vi "start.vi"() -> ()   [LabVIEW 2018]
uses:
  <vilib>/picture/picture.llb/imagedata.ctl
  SerialGlobal.vi
panel:
  out "Loop counts":i32
  out "ScanCode":i16
  out "NewVal":string
  out "Key":string
  in  "hum_pos":cluster{"pos.x":i32, "pos.y":i32}
  out "Main path":path
  out "image array":T1[](array[typedef])
  out "picture":picture
  out "status array":u8[][](array[numeric])
  in  "stage list":u32(ring) items=["stage01.map", "stage02.map", "stage03.map", "stage04.map", "stage05.map", "stage06.map", "stage07.map", "stage08.map", "stage09.map", "stage10.map", "stage11.map", "stage12.map", "stage13.map", "stage14.map", "stage15.map", "stage16.map", "stage17.map", "stage18.map", "stage19.map", "stage20.map", "stage21.map", "stage22.map", "stage23.map", "stage24.map", "stage25.map", "stage26.map", "stage27.map", "stage28.map", "stage29.map", "stage30.map", "stage31.map", "stage32.map", "stage33.map", "stage34.map", "stage35.map", "stage36.map", "stage37.map", "stage38.map", "stage39.map", "stage40.map"]
  in  "exit":bool
  in  "load stage":bool
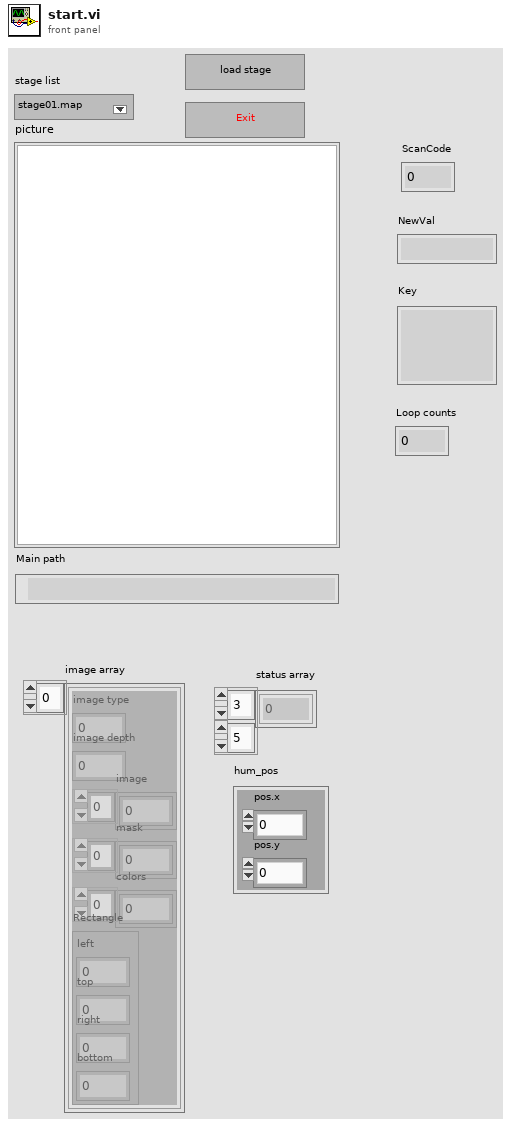
[diagram p1: front panel]
types:
  T1 = typedef "imagedata.ctl" = cluster{"image type":i32, "image depth":i32, "image":u8[], "mask":u8[], "colors":u32[], "Rectangle":cluster{"left":i16, "top":i16, "right":i16, "bottom":i16}}
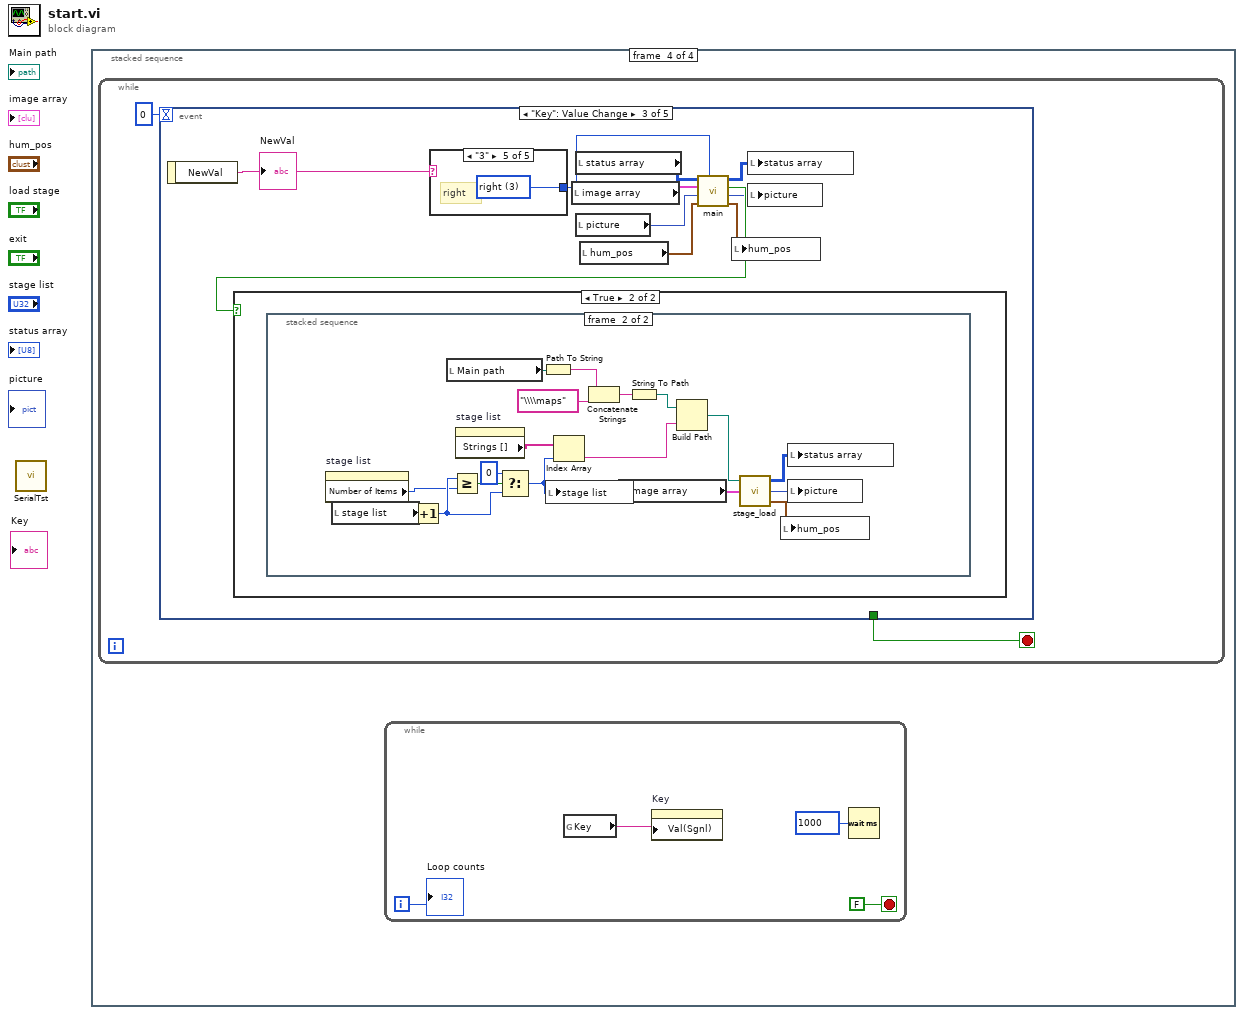
[diagram p0: block diagram]
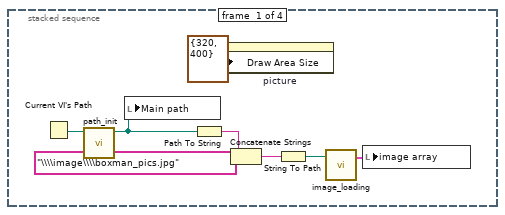
[diagram p2: hidden frame]
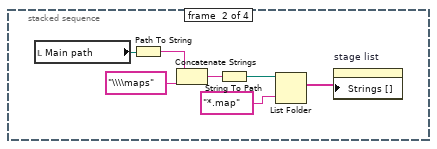
[diagram p3: hidden frame]
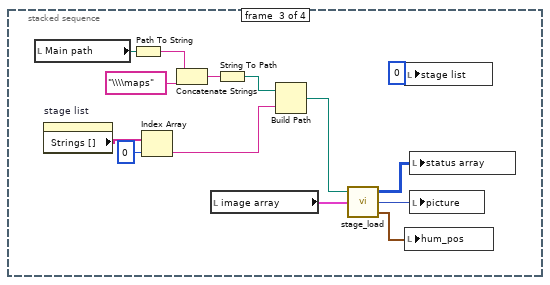
[diagram p4: hidden frame]
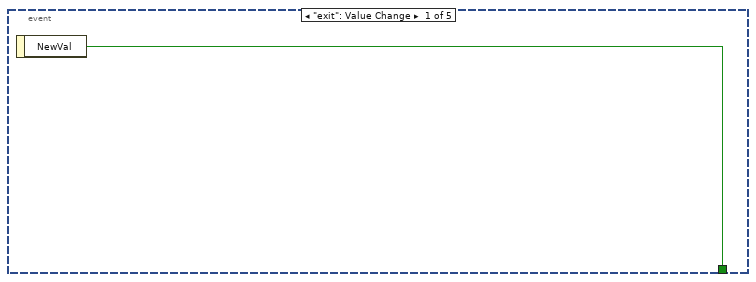
[diagram p5: hidden frame]
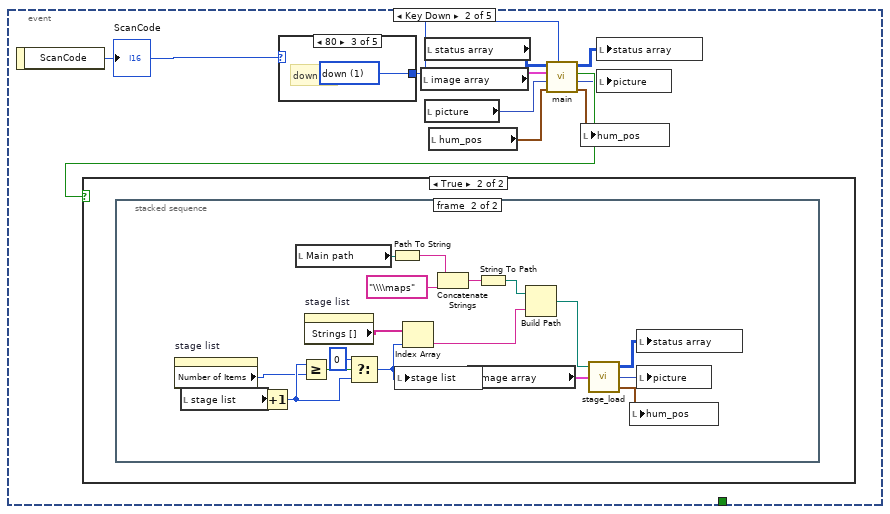
[diagram p6: hidden frame]
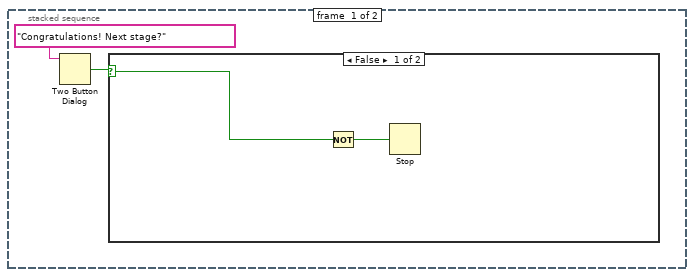
[diagram p8: hidden frame]
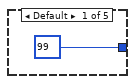
[diagram p10: hidden frame]
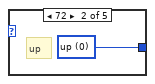
[diagram p11: hidden frame]
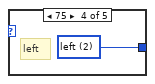
[diagram p12: hidden frame]
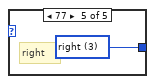
[diagram p13: hidden frame]
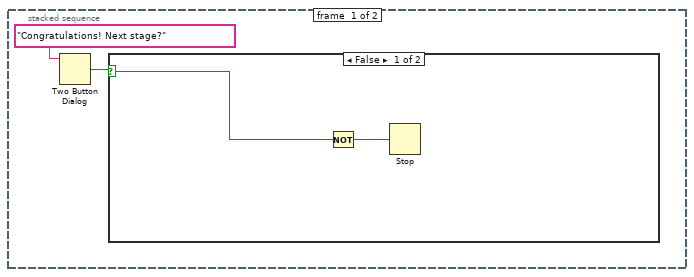
[diagram p15: hidden frame]
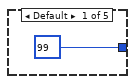
[diagram p17: hidden frame]
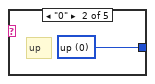
[diagram p18: hidden frame]
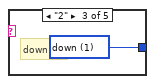
[diagram p19: hidden frame]
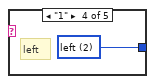
[diagram p20: hidden frame]
diagram:
  n1 = call "SerialTst.vi"() -> ()  [unwired: 12 in]
  n2 = stacked-sequence {
    frame #0 {
      n3 = Current VI's Path() -> (path=w8:path)
      n4 = call "path_init.vi"("Main vi's path"=w8) -> ("Stripped path"=w1:path)  [unwired: 5 in, 1 out]
      n5 = local write "Main path"(w1) -> ()
      n6 = Path To String(path=w1) -> (string=w5:string)
      n7 = property on="picture" class="Pict"("Draw Area Size"=cluster{"Width":u32, "Height":u32} {"Width"=320, "Height"=400}) -> ()  [unwired: 2 in, 2 out]
      n8 = Concatenate Strings(w5, "\\\\image\\\\boxman_pics.jpg" ("path to JPEG file")) -> (w4:string)
      n9 = String To Path(string=w4) -> (path=w3:path)
      n10 = call "image_loading.vi"("path to JPEG file"=w3) -> ("image array"=w7:T1[])  [unwired: 2 in]
      n11 = local write "image array"(w7) -> ()
    }
    frame #1 {
      n12 = local read "Main path"() -> (w9:path)
      n13 = Path To String(path=w9) -> (string=w14:string)
      n14 = Concatenate Strings(w14, "\\\\maps" ("path to JPEG file")) -> (w13:string)
      n15 = String To Path(string=w13) -> (path=w12:path)
      n16 = List Folder(path=w12, pattern="*.map") -> (filenames=w10:string[])  [unwired: 2 in, 3 out]
      n17 = property on="stage list" class="Ring (strict)"("Strings []"=w10) -> ()  [unwired: 2 in, 2 out]
    }
    frame #2 {
      n18 = local read "Main path"() -> (w17:path)
      n19 = property on="stage list" class="Ring (strict)"() -> ("Strings []"=w26:string[])  [unwired: 2 in, 2 out]
      n20 = Path To String(path=w17) -> (string=w23:string)
      n21 = Index Array(array=w26, index=0) -> (element=w22:string)
      n22 = Concatenate Strings(w23, "\\\\maps" ("path to JPEG file")) -> (w21:string)
      n23 = local read "image array"() -> (w29:T1[])
      n24 = String To Path(string=w21) -> (path=w20:path)
      n25 = Build Path(base path=w20, name or relative path=w22) -> (appended path=w19:path)
      n26 = call "stage_load.vi"("image array"=w29, "map file"=w19) -> ("hum_pos"=w16:cluster{"pos.x":i32, "pos.y":i32}, "picture"=w27:picture, "status array"=w28:u8[][])  [unwired: 1 in]
      n27 = local write "stage list"(0) -> ()
      n28 = local write "hum_pos"(w16) -> ()
      n29 = local write "status array"(w28) -> ()
      n30 = local write "picture"(w27) -> ()
    }
    frame #3 {
      n31 = while {
        stop <- w35 stop-if-true
        n32 = event shown="[2] \"Key\": Value Change" {
          selector: _ -> [_ _ _ _ _]
          dyn-events: _ -> [_ _ _ _ _]
          timeout: 0 -> [_ _ _ _ _]
          tunnel: [w36 _ _ _ _] -> w35
          event "exit": Value Change {
            n33 = event-data() -> ("NewVal"=w36:bool)  [unwired: 1 in]
          }
          event Key Down {
            n34 = event-data() -> ("ScanCode"=w37:i16)  [unwired: 1 in]
            "ScanCode" <- w37
            n35 = case shown="80" w37 {
              tunnel: [u8 99 ("function") w70 w71 w72 w73] -> w44
              frame Default {
              }
              frame 72 {
                w70 = u8 0 items=["up", "down", "left", "right"] ("function")
                # "up"
              }
              frame 80 {
                w71 = u8 1 items=["up", "down", "left", "right"] ("function")
                # "down"
              }
              frame 75 {
                w72 = u8 2 items=["up", "down", "left", "right"] ("function")
                # "left"
              }
              frame 77 {
                w73 = u8 3 items=["up", "down", "left", "right"] ("function")
                # "right"
              }
            }
            n36 = local read "image array"() -> (w42:T1[])
            n37 = local read "status array"() -> (w45:u8[][])
            n38 = local read "picture"() -> (w41:picture)
            n39 = local read "hum_pos"() -> (w40:cluster{"pos.x":i32, "pos.y":i32})
            n40 = call "main.vi"("function"=w44, "hum_pos in"=w40, "picture in"=w41, "image array"=w42, "status array in"=w45) -> ("hum_pos out"=w39:cluster{"pos.x":i32, "pos.y":i32}, "picture out"=w38:picture, "stage pass?"=w43:bool, "status array out"=w46:u8[][])
            n41 = case shown="True" w43 {
              frame False {
              }
              frame True {
                n42 = stacked-sequence {
                  frame #0 {
                    n43 = Two Button Dialog(message="Congratulations! Next stage?") -> (T button?=w47:bool)  [unwired: 2 in]
                    n44 = case shown="False" w47 {
                      selector: w47 -> [w49 _]
                      frame False {
                        n45 = Not(x=w49) -> (.not. x?=w50:bool)
                        n46 = Stop(stop? (T)=w50) -> ()
                      }
                      frame True {
                      }
                    }
                  }
                  frame #1 {
                    n47 = property on="stage list" class="Ring (strict)"() -> ("Number of Items"=w54:u32)  [unwired: 2 in, 2 out]
                    n48 = local read "stage list"() -> (w53:u32)
                    n49 = Increment(x=w53) -> (x+1=w57:u32)
                    n50 = local read "Main path"() -> (w58:path)
                    n51 = Greater Or Equal?(x=w57, y=w54) -> (x >= y?=w55:bool)
                    n52 = property on="stage list" class="Ring (strict)"() -> ("Strings []"=w65:string[])  [unwired: 2 in, 2 out]
                    n53 = Select(t=0, s=w55, f=w57) -> (s? t:f=w52:u32)
                    n54 = Path To String(path=w58) -> (string=w63:string)
                    n55 = local write "stage list"(w52) -> ()
                    n56 = Index Array(array=w65, index=w52) -> (element=w62:string)
                    n57 = Concatenate Strings(w63, "\\\\maps" ("path to JPEG file")) -> (w61:string)
                    n58 = local read "image array"() -> (w68:T1[])
                    n59 = String To Path(string=w61) -> (path=w60:path)
                    n60 = Build Path(base path=w60, name or relative path=w62) -> (appended path=w59:path)
                    n61 = call "stage_load.vi"("image array"=w68, "map file"=w59) -> ("hum_pos"=w51:cluster{"pos.x":i32, "pos.y":i32}, "picture"=w66:picture, "status array"=w67:u8[][])  [unwired: 1 in]
                    n62 = local write "hum_pos"(w51) -> ()
                    n63 = local write "status array"(w67) -> ()
                    n64 = local write "picture"(w66) -> ()
                  }
                }
              }
            }
            n65 = local write "hum_pos"(w39) -> ()
            n66 = local write "status array"(w46) -> ()
            n67 = local write "picture"(w38) -> ()
          }
          event "Key": Value Change {
            n68 = event-data() -> ("NewVal"=w74:string)  [unwired: 1 in]
            "NewVal" <- w74
            n69 = case shown="\"3\"" w74 {
              tunnel: [u8 99 ("function") w107 w108 w109 w110] -> w81
              frame Default {
              }
              frame "0" {
                w107 = u8 0 items=["up", "down", "left", "right"] ("function")
                # "up"
              }
              frame "2" {
                w108 = u8 1 items=["up", "down", "left", "right"] ("function")
                # "down"
              }
              frame "1" {
                w109 = u8 2 items=["up", "down", "left", "right"] ("function")
                # "left"
              }
              frame "3" {
                w110 = u8 3 items=["up", "down", "left", "right"] ("function")
                # "right"
              }
            }
            n70 = local read "image array"() -> (w79:T1[])
            n71 = local read "status array"() -> (w82:u8[][])
            n72 = local read "picture"() -> (w78:picture)
            n73 = local read "hum_pos"() -> (w77:cluster{"pos.x":i32, "pos.y":i32})
            n74 = call "main.vi"("function"=w81, "hum_pos in"=w77, "picture in"=w78, "image array"=w79, "status array in"=w82) -> ("hum_pos out"=w76:cluster{"pos.x":i32, "pos.y":i32}, "picture out"=w75:picture, "stage pass?"=w80:bool, "status array out"=w83:u8[][])
            n75 = case shown="True" w80 {
              frame False {
              }
              frame True {
                n76 = stacked-sequence {
                  frame #0 {
                    n77 = Two Button Dialog(message="Congratulations! Next stage?") -> (T button?=w84:bool)  [unwired: 2 in]
                    n78 = case shown="False" w84 {
                      selector: w84 -> [w86 _]
                      frame False {
                        n79 = Not(x=w86) -> (.not. x?=w87:bool)
                        n80 = Stop(stop? (T)=w87) -> ()
                      }
                      frame True {
                      }
                    }
                  }
                  frame #1 {
                    n81 = property on="stage list" class="Ring (strict)"() -> ("Number of Items"=w91:u32)  [unwired: 2 in, 2 out]
                    n82 = local read "stage list"() -> (w90:u32)
                    n83 = Increment(x=w90) -> (x+1=w94:u32)
                    n84 = local read "Main path"() -> (w95:path)
                    n85 = Greater Or Equal?(x=w94, y=w91) -> (x >= y?=w92:bool)
                    n86 = property on="stage list" class="Ring (strict)"() -> ("Strings []"=w102:string[])  [unwired: 2 in, 2 out]
                    n87 = Select(t=0, s=w92, f=w94) -> (s? t:f=w89:u32)
                    n88 = Path To String(path=w95) -> (string=w100:string)
                    n89 = local write "stage list"(w89) -> ()
                    n90 = Index Array(array=w102, index=w89) -> (element=w99:string)
                    n91 = Concatenate Strings(w100, "\\\\maps" ("path to JPEG file")) -> (w98:string)
                    n92 = local read "image array"() -> (w105:T1[])
                    n93 = String To Path(string=w98) -> (path=w97:path)
                    n94 = Build Path(base path=w97, name or relative path=w99) -> (appended path=w96:path)
                    n95 = call "stage_load.vi"("image array"=w105, "map file"=w96) -> ("hum_pos"=w88:cluster{"pos.x":i32, "pos.y":i32}, "picture"=w103:picture, "status array"=w104:u8[][])  [unwired: 1 in]
                    n96 = local write "hum_pos"(w88) -> ()
                    n97 = local write "status array"(w104) -> ()
                    n98 = local write "picture"(w103) -> ()
                  }
                }
              }
            }
            n99 = local write "hum_pos"(w76) -> ()
            n100 = local write "status array"(w83) -> ()
            n101 = local write "picture"(w75) -> ()
          }
          event "load stage": Value Change {
            n102 = event-data() -> ("NewVal"=w111:bool)  [unwired: 1 in]
            n103 = case shown="True" w111 {
              frame False {
              }
              frame True {
                n104 = local read "Main path"() -> (w113:path)
                n105 = local read "stage list"() -> (w125:u32)
                n106 = property on="stage list" class="Ring (strict)"() -> ("Strings []"=w121:string[])  [unwired: 2 in, 2 out]
                n107 = Path To String(path=w113) -> (string=w119:string)
                n108 = Index Array(array=w121, index=w125) -> (element=w118:string)
                n109 = Concatenate Strings(w119, "\\\\maps" ("path to JPEG file")) -> (w117:string)
                n110 = local read "image array"() -> (w124:T1[])
                n111 = String To Path(string=w117) -> (path=w116:path)
                n112 = Build Path(base path=w116, name or relative path=w118) -> (appended path=w115:path)
                n113 = call "stage_load.vi"("image array"=w124, "map file"=w115) -> ("hum_pos"=w112:cluster{"pos.x":i32, "pos.y":i32}, "picture"=w122:picture, "status array"=w123:u8[][])  [unwired: 1 in]
                n114 = local write "load stage"(FALSE) -> ()
                n115 = local write "hum_pos"(w112) -> ()
                n116 = local write "status array"(w123) -> ()
                n117 = local write "picture"(w122) -> ()
              }
            }
          }
          event Timeout {
            n118 = event-data() -> ()  [unwired: 1 in, 3 out]
          }
        }
      }
      n119 = while {
        i -> [w31]
        stop <- FALSE stop-if-true
        n120 = global read "SerialGlobal.vi" "Key"() -> (w33:string)
        n121 = property on="Key" class="Str"("Val(Sgnl)"=w33) -> ()  [unwired: 2 in, 2 out]
        n122 = Wait (ms)(milliseconds to wait=u32 1000) -> ()  [unwired: 1 out]
        "Loop counts" <- w31
      }
    }
  }
